vi "Check Timeout.vi"(4 "Timeout Expected(ms)":i32=100, 8 "Force Timeout?":bool) -> (3 "Timeout":bool)   [LabVIEW 2017, in "csm-tool-support.lvlib"]
doc: "Used in templates with a user event structure.\n\n-- <b>Controls</b> --\n- <b>Timeout Expected</b>: Expected timeout setting\n- <b>Remaining States</b>: Outputs 0 if there are remaining states; otherwise, outputs the expected value\n\n-- <b>Indicators</b> --\n- <b>Timeout</b>: Timeout setting after arbitration"
uses:
  csm-tool-support.lvlib
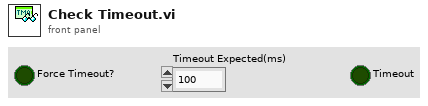
[diagram p1: front panel]
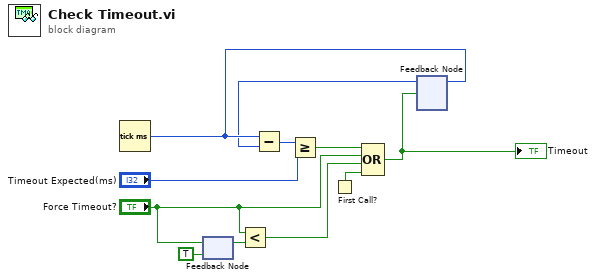
[diagram p0: block diagram]
diagram:
  n1 = Tick Count (ms)() -> (millisecond timer value=w9:u32)
  n2 = feedback #1(TRUE ("Force Timeout?")) -> (w4:bool)
  n3 = feedback-in #1("Force Timeout?") -> ()
  n4 = Less?(x="Force Timeout?", y=w4) -> (x < y?=w2:bool)
  n5 = First Call?() -> (First Call?: T/F=w1:bool)
  n6 = feedback #2() -> (w6:u32)  [unwired: 1 in]
  n7 = Subtract(x=w9, y=w6) -> (x-y=w8:u32)
  n8 = Greater Or Equal?(x=w8, y="Timeout Expected(ms)") -> (x >= y?=w7:bool)
  n9 = Compound Arithmetic op=OR(w7, "Force Timeout?", w2, w1) -> (w10:bool)
  "Timeout" <- w10
  n10 = feedback-in #2(w9, w10) -> ()
